vi "MPURequest.vi"(0 "FIFO":refnum<k21>) -> ()   [LabVIEW 2018]
uses:
  <vilib>/rvi/DataTransferAndStorage/Container/Common/niFpgaContainerExecOnDevCompGetState.vi
  <vilib>/rvi/Emulation/niFpgaEmulationIsFPGAContextNoSignature.vi
  <vilib>/rvi/Emulation/niFpgaSctlEmulationGetInTimedLoop.vi
  <vilib>/rvi/errors/niFpgaSetErrorForExecOnDevCompSimple.vi
  <vilib>/rvi/eio/common/nirviEmuReportErrorAndStop.vi
  <vilib>/rvi/DataTransferAndStorage/Container/Common/niFpgaContainerGetUniqueNameForEmu.vi
  <vilib>/rvi/FIFO/Fifo_Resource/nirvififoEmulationSetSize.vi
  <vilib>/rvi/FIFO/Fifo_Resource/nirviFifoEmulationQueueMgr.vi
  <instcachedir>/0/nirviFifoEmulationQueueMgr_E5CAEC123FF24DC58D834DCA3CDAA9B5.lvgen/nirviFifoEmulationQueueMgr_E5CAEC123FF24DC58D834DCA3CDAA9B5_001.vi
  <vilib>/rvi/FIFO/Fifo_Resource/nirvififoEmulationDetermineInputValidOut.vi
  <vilib>/rvi/FIFO/Fifo_Resource/nirvififoEmulationCreateLock.vi
  <vilib>/rvi/Emulation/niFpgaProcessEmulError.vi
  <vilib>/rvi/FIFO/Fifo_Resource/nirvififoEmulationObtainLock.vi
  <vilib>/rvi/FIFO/Fifo_Resource/nirvififoEmulationReleaseLock.vi
  <vilib>/rvi/occurrence/nirviWaitOnOccurrenceBase.vi
  <vilib>/rvi/errors/nirviReportUnexpectedCaseInternalError.vi
  <vilib>/rvi/errors/nirviReportUnexpectedCaseInternalError (U32).vi
  <vilib>/Utility/error.llb/Clear Errors.vi
  <vilib>/rvi/interface/RandomDataEmulation/niFpgaRandomDataHandleErrors.vi
  <vilib>/rvi/DataTransferAndStorage/Container/XNode/niFpgaContainer.xnode
  <vilib>/rvi/FIFO/Fifo_Resource/niFpgaFifoEmulationRefIn.vi
  <vilib>/rvi/interface/RandomDataEmulation/nirviRandomDataFpgaReadWriteTemplate.vi
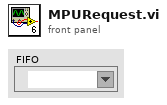
[diagram p1: front panel]
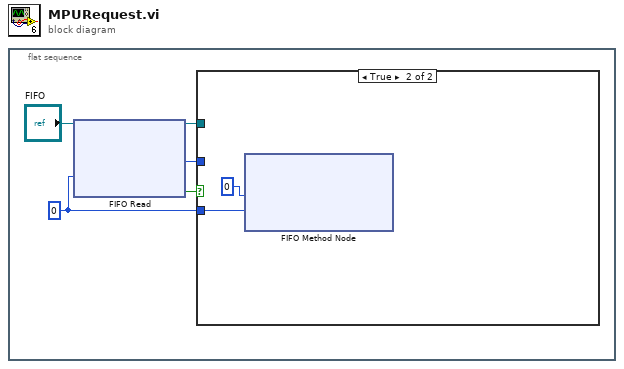
[diagram p0: block diagram]
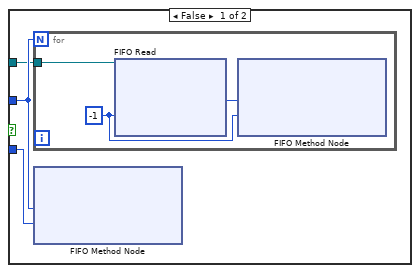
[diagram p2: hidden frame]
diagram:
  n1 = flat-sequence {
    frame #0 {
      w4 = 0 ("Timeout")
      n2 = xnode "FIFO Read"("Timeout"=w4, "FIFO In"="FIFO") -> ("Element"=w3:u8, "Timed Out?"=w1:bool, "FIFO Out"=w2:refnum<k21>)
      n3 = case shown="True" w1 {
        tunnel: w4 -> [w8 w13]
        tunnel: w3 -> [w7 _]
        tunnel: w2 -> [w6 _]
        frame False {
          n4 = for {
            N: w7 -> [_]
            tunnel: w6 -> [w11]
            w9 = -1 ("Timeout")
            n5 = xnode "FIFO Read"("Timeout"=w9, "FIFO In"=w11) -> ("Element"=w10:u8)  [unwired: 2 out]
            n6 = xnode ("FIFO Method Node")("Element"=w10, "Timeout"=w9) -> ()  [unwired: 1 in, 2 out]
          }
          n7 = xnode ("FIFO Method Node")("Element"=w7, "Timeout"=w8) -> ()  [unwired: 1 in, 2 out]
        }
        frame True {
          n8 = xnode ("FIFO Method Node")("Element"=u8 0, "Timeout"=w13) -> ()  [unwired: 1 in, 2 out]
        }
      }
    }
  }
